vi "SetTemperatureRange(SubVI).vi"(9 "Temperature Range (Low) in":dbl, 10 "Temperature Range (High) in":dbl, 11 "Refnum in":refnum<k35>) -> ()   [LabVIEW 2020]
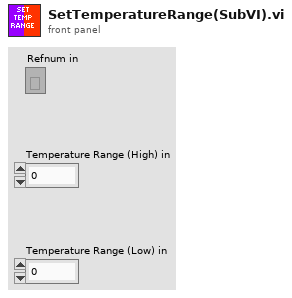
[diagram p1: front panel]
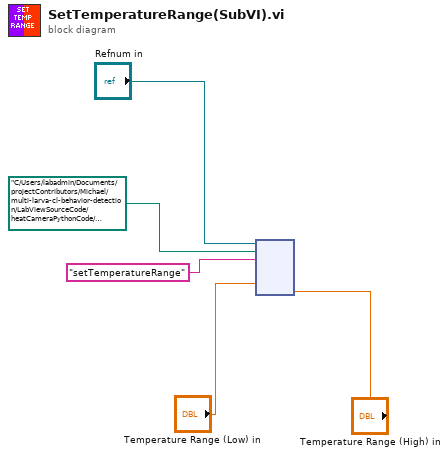
[diagram p0: block diagram]
diagram:
  n1 = node("Refnum in", path "C:/Users/labadmin/Documents/projectContributors/Michael/multi-larva-cl-behavior-detection/LabViewSourceCode/heatCameraPythonCode/customFlir.py" ("module path"), "setTemperatureRange" ("function name"), "Temperature Range (Low) in", "Temperature Range (High) in") -> ()  [unwired: 5 in, 4 out]
